vi "Read Builld Path.vi"(9 "PythonConverter_GUI in":refnum<class "PythonConverter_GUI.lvclass">) -> (3 "PythonConverter_GUI out":refnum<class "PythonConverter_GUI.lvclass">, 4 "Builld Path":path)   [LabVIEW 2014, in "PythonConverter_GUI.lvclass"]
uses:
  PythonConverter_GUI.lvclass
  PythonConverter_GUI.lvclass/PythonConverter_GUI.ctl
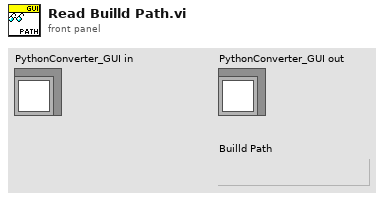
[diagram p1: front panel]
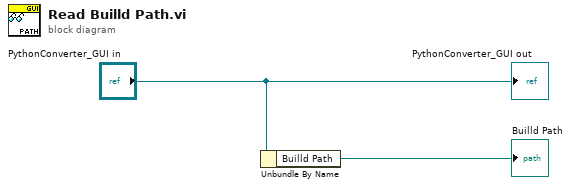
[diagram p0: block diagram]
diagram:
  n1 = Unbundle By Name("PythonConverter_GUI in") -> ("Builld Path"=→"Builld Path":path)
  "PythonConverter_GUI out" <- "PythonConverter_GUI in"
